vi "Initialize.vi"(8 "error in (no error)":errorcluster, 9 "ID Query":bool, 10 "Reset":bool, 11 "Generic Power Analyzer in":refnum<class "Generic Power Analyzer.lvclass">) -> (0 "error out":errorcluster, 2 "VISA resource name":refnum<visa-resource-name>, 3 "Generic Power Analyzer out":refnum<class "Generic Power Analyzer.lvclass">)   [LabVIEW 2014, in "Generic Power Analyzer.lvlib" / "Generic Power Analyzer.lvclass"]
uses:
  Generic Power Analyzer.lvclass
  Abstract Sensor/Abstract Sensor.lvclass
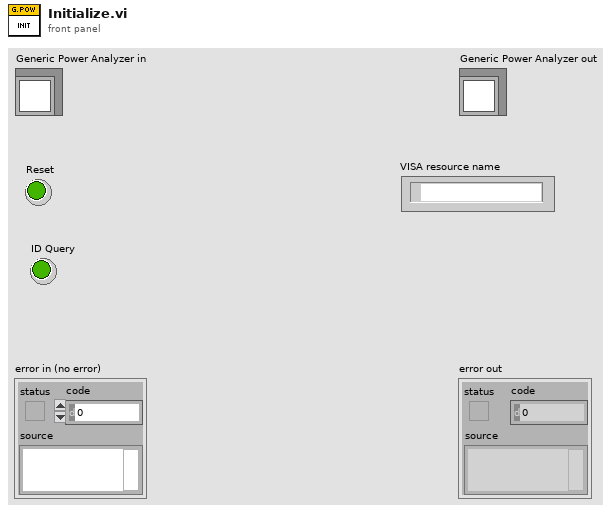
[diagram p1: front panel]
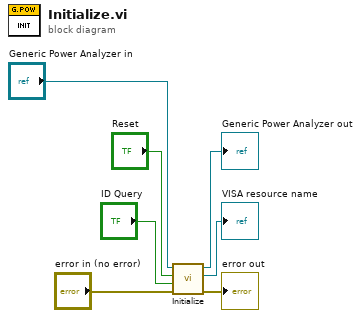
[diagram p0: block diagram]
diagram:
  n1 = call-parent "Initialize.vi"("error in (no error)"="error in (no error)", "ID Query"="ID Query", "Reset"="Reset", "Abstract Sensor in"="Generic Power Analyzer in") -> ("error out"=→"error out":errorcluster, "VISA resource name"=→"VISA resource name":refnum<visa-resource-name>, "Abstract Sensor out"=→"Generic Power Analyzer out":refnum<class "Generic Power Analyzer.lvclass">)  [unwired: 5 in]
